vi "Read Actor ID.vi"(11 "Monitored Actor in":refnum<class "Monitored Actor.lvclass">) -> (2 "Actor ID":string, 3 "Monitored Actor out":refnum<class "Monitored Actor.lvclass">)   [LabVIEW 2018, in "Monitored Actor.lvlib" / "Monitored Actor.lvclass"]
doc: "Reads the Actor's ID\n\nCopyright: MGI\nAuthored by: Derek Trepanier"
uses:
  Monitored Actor.lvclass
  Monitored Actor.lvclass/Monitored Actor.ctl
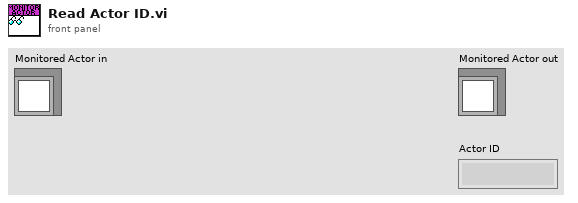
[diagram p1: front panel]
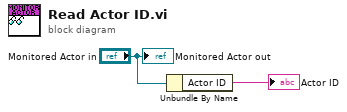
[diagram p0: block diagram]
diagram:
  n1 = Unbundle By Name("Monitored Actor in") -> ("Actor ID"=→"Actor ID":string)
  "Monitored Actor out" <- "Monitored Actor in"
